vi "RT Driver.vi"(7 "Operation":T1, 11 "Device Reference in":T2 format="%.0x") -> (0 "Error Code":i32)   [LabVIEW 2012, in "PXImc Engine.lvlib"]
uses:
  PXImc Engine.lvlib
  <vilib>/NI Veristand/Custom Device API/Custom Device Item Ref.ctl
  <vilib>/NI Veristand/Custom Device API/Hardware Interface Driver VI Operation.ctl
  RT Data Cluster.ctl
  Shared/Compiled Data.ctl
  <vilib>/NI Veristand/Custom Device API/Block Data Reference.ctl
  <vilib>/NI Veristand/Custom Device API/Data Reference.ctl
  Shared/PXImc Shared.lvlib
  <vilib>/NI Veristand/Custom Device API/Custom Device API.lvlib
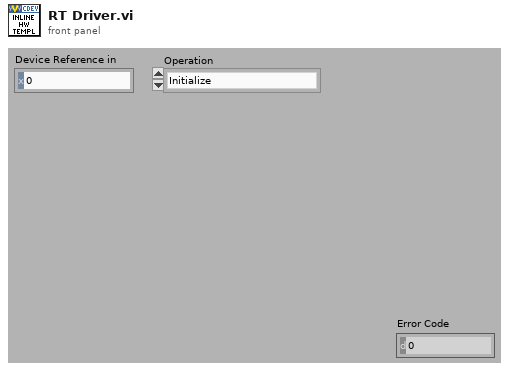
[diagram p1: front panel]
types:
  T1 = typedef "Custom Device API.lvlib/Hardware Interface Driver VI Operation.ctl" = enum16{"Initialize", "Start", "Read Data from HW", "Write Data to HW", "Close"}
  T2 = typedef "Custom Device API.lvlib/Custom Device Item Ref.ctl" = u64
  T3 = typedef "PXImc Engine.lvlib/RT Data Cluster.ctl" = cluster{"Compiled Data":T4, "Read Session":refnum<k21>, "Write Session":refnum<k21>, "SendRefs":T5[], "SendVals":dbl[], "ReceiveRefs":T5[], "StatusRefs":T6[], "RFull Count":dbl, "#toRead":i32, "#toWrite":i32, "WLate Count":dbl, "ReadBufSize":i32, "RLow Count":dbl}
  T4 = typedef "PXImc Shared.lvlib/Compiled Data.ctl" = cluster{"My write ID":u16, "Remote write ID":u16, "Module Name":string, "Name":string}
  T5 = typedef "Custom Device API.lvlib/Block Data Reference.ctl" = cluster{"Data Reference":T6, "Offset":i32, "Length":i32}
  T6 = typedef "Custom Device API.lvlib/Data Reference.ctl" = i32
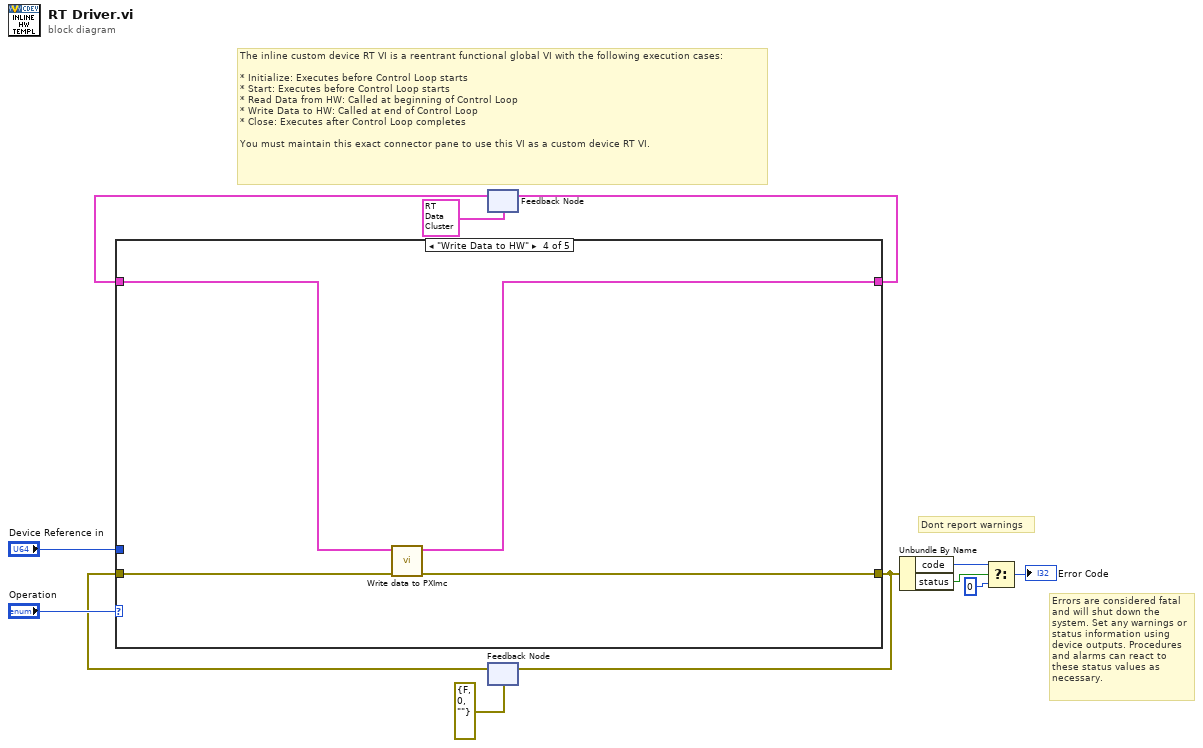
[diagram p0: block diagram]
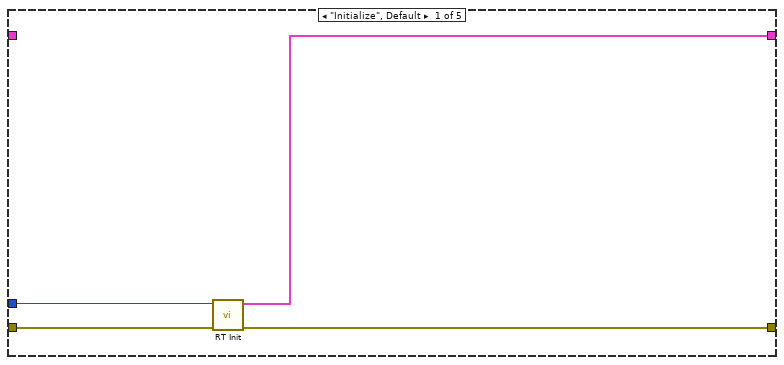
[diagram p2: hidden frame]
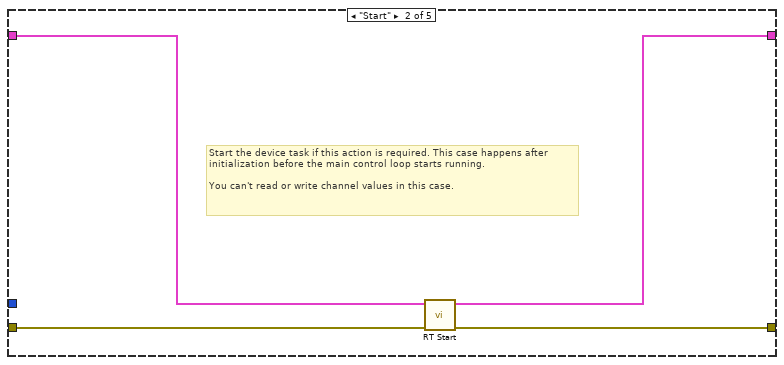
[diagram p3: hidden frame]
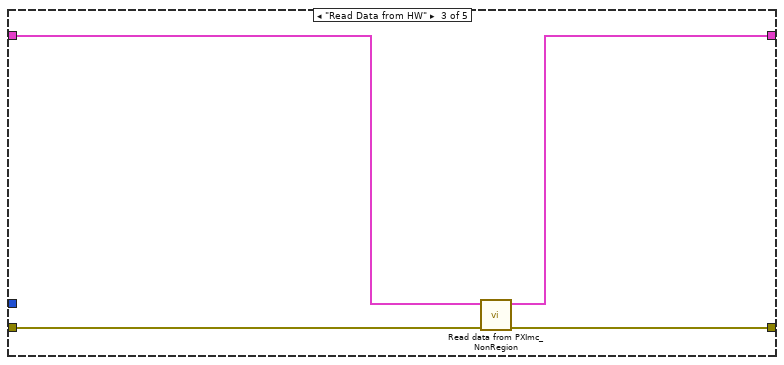
[diagram p4: hidden frame]
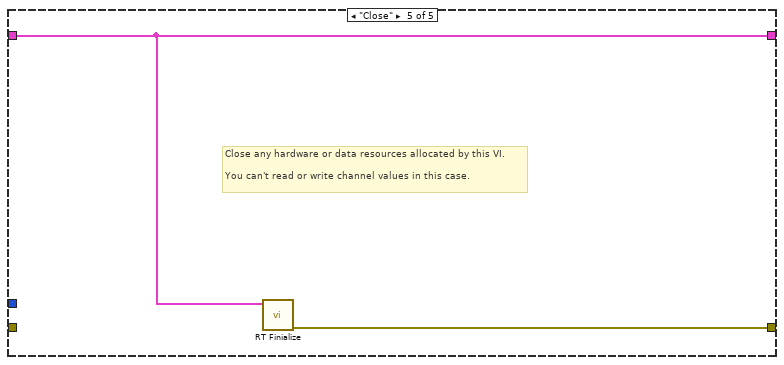
[diagram p5: hidden frame]
diagram:
  # "Dont report warnings"
  # "Errors are considered fatal and will shut down the system. Set any warnings or status information using device outputs. Procedures and alarms can react to these status values as necessary."
  # "The inline custom device RT VI is a reentrant functional global VI with the following execution cases:\n\n* Initialize: Executes before Control Loop starts\n* Start: Executes before Control Loop starts\n* Read Data from HW: Called at beginning of Control Loop\n* Write Data to HW: Called at end of Control Loop\n* Close: Executes after Control Loop completes\n\nYou must maintain this exact connector pane to use this VI as a custom device RT VI."
  n1 = feedback #1(T3 {"Compiled Data"={"My write ID"=0, "Remote write ID"=0, "Module Name"="", "Name"=""}, "Read Session"="", "Write Session"="", "SendRefs"=[], "SendVals"=[], "ReceiveRefs"=[], "StatusRefs"=[], "RFull Count"=0.0, "#toRead"=0, "#toWrite"=0, "WLate Count"=0.0, "ReadBufSize"=0, "RLow Count"=0.0} ("RT Data Cluster")) -> (w10:T3)
  n2 = feedback #2(errorcluster {"status"=FALSE, "code"=0, "source"=""} ("error constant")) -> (w2:errorcluster)
  n3 = case shown="\"Write Data to HW\"" "Operation" {
    tunnel: [w15 w18 w23 w26 w30] -> w11
    tunnel: w10 -> [_ w19 w24 w27 w30]
    tunnel: "Device Reference in" -> [w16 _ _ _ _]
    tunnel: [w14 w17 w21 w25 w29] -> w3
    tunnel: w2 -> [w13 w20 w22 w28 _]
    frame "Initialize", Default {
      n4 = call "RT Init.vi"("error in"=w13, "Device Ref"=w16) -> ("error out"=w14:errorcluster, "RT Data"=w15:T3)  [unwired: 8 in]
    }
    frame "Start" {
      # "Start the device task if this action is required. This case happens after initialization before the main control loop starts running.\n\nYou can't read or write channel values in this case."
      n5 = call "RT Start.vi"("error in (no error)"=w20, "RT Data Cluster in"=w19) -> ("error out"=w17:errorcluster, "RT Data Cluster out"=w18:T3)  [unwired: 8 in]
    }
    frame "Read Data from HW" {
      n6 = call "Read data from PXImc_NonRegion.vi"("error in (no error)"=w22, "RT Data Cluster in"=w24) -> ("error out"=w21:errorcluster, "RT Data Cluster out"=w23:T3)  [unwired: 8 in]
    }
    frame "Write Data to HW" {
      n7 = call "Write data to PXImc.vi"("error in (no error)"=w28, "RT Data Cluster in"=w27) -> ("error out"=w25:errorcluster, "RT Data Cluster out"=w26:T3)  [unwired: 8 in]
    }
    frame "Close" {
      # "Close any hardware or data resources allocated by this VI.\n\nYou can't read or write channel values in this case."
      n8 = call "RT Finialize.vi"("RT Data Cluster in"=w30) -> ("error out"=w29:errorcluster)  [unwired: 10 in]
    }
  }
  n9 = feedback-in #1(w11) -> ()
  n10 = feedback-in #2(w3) -> ()
  n11 = Unbundle By Name(w3) -> ("code"=w6:i32, "status"=w7:bool)
  n12 = Select(t=w6, s=w7, f=0) -> (s? t:f=→"Error Code":i32)
